vi "Config dialog.vi"(8 "error in (no error)":errorcluster, 11 "Device Name in":tag) -> (0 "error out":errorcluster, 2 "Cancelled?":bool, 3 "Device Name out":tag)   [LabVIEW 2020]
uses:
  Config states ---typedef.ctl
  <resource>/objmgr/daqmx.rc
panel:
  in  "Device Name":tag
  in  "Cancel Button":bool
  in  "OK Button":bool
  out "Modelo":string
  out "Serial":u32 caption="# de serie"
  in  "Test device":bool
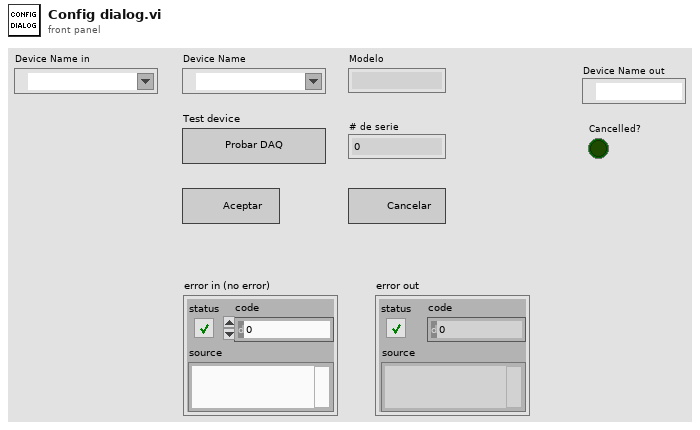
[diagram p1: front panel]
types:
  T1 = typedef "Config states ---typedef.ctl" = enum16{"Init", "Wait", "Exit"}
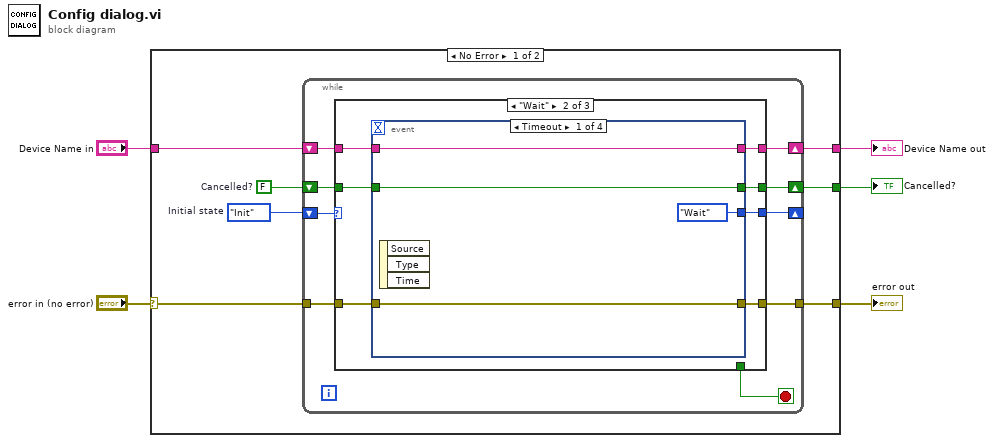
[diagram p0: block diagram]
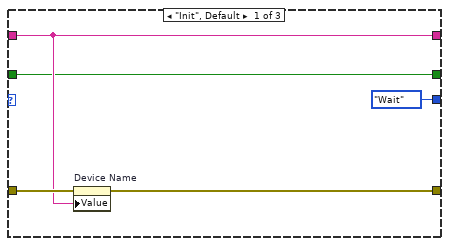
[diagram p2: hidden frame]
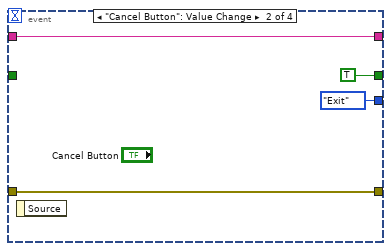
[diagram p3: hidden frame]
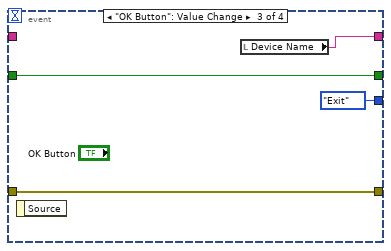
[diagram p4: hidden frame]
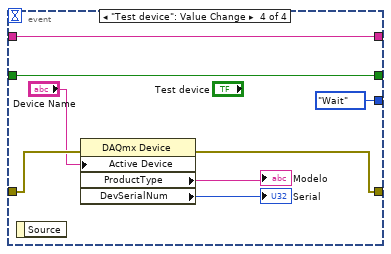
[diagram p5: hidden frame]
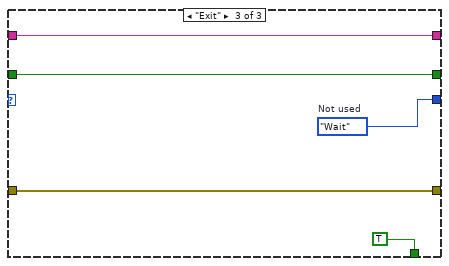
[diagram p6: hidden frame]
diagram:
  n1 = case shown="No Error" "error in (no error)" {
    selector: "error in (no error)" -> [w10 w60]
    tunnel: "Device Name in" -> [w12 w59]
    tunnel: [w11 w59] -> w4
    tunnel: [w9 w60] -> w2
    tunnel: [w8 _] -> w1
    frame No Error {
      w6 = FALSE  # Cancelled?
      w7 = Config_states_---typedef."Init"  # Initial state
      n2 = while {
        shift-right: [w20] -> _
        shift-left: w7 -> [w21]
        shift-right: [w18] -> w11
        shift-left: w12 -> [w19]
        tunnel: w10 -> [w17]
        tunnel: [w16] -> w9
        shift-right: [w14] -> w8
        shift-left: w6 -> [w13]
        stop <- w15 stop-if-true
        n3 = case shown="\"Wait\"" w21 {
          tunnel: [Config_states_---typedef."Wait" w33 w55] -> w20
          tunnel: w19 -> [w23 w30 w58]
          tunnel: [w23 w29 w58] -> w18
          tunnel: w17 -> [w25 w32 w57]
          tunnel: [w24 w31 w57] -> w16
          tunnel: [_ _ TRUE] -> w15
          tunnel: [w22 w28 w54] -> w14
          tunnel: w13 -> [w22 w27 w54]
          frame "Init", Default {
            n4 = property on="Device Name" class="DAQmxName"(error in=w25, "Value"=w23) -> (error out=w24:errorcluster)  [unwired: 1 in, 1 out]
          }
          frame "Wait" {
            n5 = event shown="[0] Timeout" {
              selector: _ -> [_ _ _ _]
              dyn-events: _ -> [_ _ _ _]
              timeout: _ -> [_ _ _ _]
              tunnel: [Config_states_---typedef."Wait" Config_states_---typedef."Exit" Config_states_---typedef."Exit" Config_states_---typedef."Wait"] -> w33
              tunnel: w32 -> [w36 w41 w45 w53]
              tunnel: [w36 w41 w45 w49] -> w31
              tunnel: w30 -> [w35 w40 _ w52]
              tunnel: [w35 w40 w44 w52] -> w29
              tunnel: [w34 TRUE w42 w46] -> w28
              tunnel: w27 -> [w34 _ w42 w46]
              event Timeout {
                n6 = event-data() -> ()  [unwired: 1 in, 3 out]
              }
              event "Cancel Button": Value Change {
                n7 = event-data() -> ()  [unwired: 1 in, 1 out]
              }
              event "OK Button": Value Change {
                n8 = event-data() -> ()  [unwired: 1 in, 1 out]
                n9 = local read "Device Name"() -> (w44:tag)
              }
              event "Test device": Value Change {
                n10 = event-data() -> ()  [unwired: 1 in, 1 out]
                n11 = property class="DAQmx Device"(error in=w53, "Active Device"="Device Name") -> (error out=w49:errorcluster, "ProductType"=→"Modelo":string, "DevSerialNum"=→"Serial":u32)  [unwired: 1 in, 1 out]
              }
            }
          }
          frame "Exit" {
            w55 = Config_states_---typedef."Wait"  # Not used
          }
        }
      }
    }
    frame Error {
    }
  }
  "Device Name out" <- w4
  "error out" <- w2
  "Cancelled?" <- w1
